vi "strain_test.vi"() -> ()   [LabVIEW 2014]
uses:
  <vilib>/LabVIEW Targets/FPGA/cRIO/shared/nicrio_ModuleControls/nicrio_cRIO-9237_ExcitationVoltageRing.ctl
  <vilib>/LabVIEW Targets/FPGA/cRIO/shared/nicrio_ModuleControls/nicrio_cRIO-9237_DataRatesRing.ctl
  <vilib>/rvi/Emulation/niFpgaGetClockAttributes.vi
  <vilib>/rvi/Emulation/niFpgaSctlEmulationGetInTimedLoop.vi
  <vilib>/rvi/Emulation/niFpgaEmulationReportErrorSimple.vi
  <vilib>/rvi/eio/common/nirviEmuTemplateMethod_errors.vi
  <vilib>/rvi/eio/common/nirviEmuTemplatePropertySet_errors.vi
  <vilib>/rvi/Emulation/niFpgaCriticalErrorInLSC.vi
  <vilib>/eio/EIONode/EIONode.xnode
  <vilib>/rvi/Analysis/measure/butterworth/XNode/niFpgaButterworthFilter.xnode
  <vilib>/eio/EIOPropertyNode/EIOPropertyNode.xnode
  <vilib>/rvi/eio/common/nirviEmuTemplatePropertyGet_errors.vi
  <vilib>/rvi/eio/common/nirviEmuTemplatePropertyGet_noerrors.vi
  <vilib>/rvi/eio/common/nirviEmuTemplatePropertySet_noerrors.vi
panel:
  in  "Offset Cal Enable":bool
  in  "Mod6/Start":bool
  out "Mod1*GF":fxp<+/-,40,9>
  out "Mod1/AI0":fxp<+/-,20,5>
  in  "Data Rate":T1=1 items=["50.000 kS/s (NI 9237)"=1, "25.000 kS/s (NI 9237)"=2, "16.667 kS/s (NI 9237)"=3, "12.500 kS/s (NI 9237)"=4, "10.000 kS/s (NI 9237)"=5, "8.333 kS/s (NI 9237)"=6, "7.143 kS/s (NI 9237)"=7, "6.250 kS/s (NI 9237)"=8, "5.556 kS/s (NI 9237)"=9, "5.000 kS/s (NI 9237)"=10, "4.545 kS/s (NI 9237)"=11, "4.167 kS/s (NI 9237)"=12, "3.846 kS/s (NI 9237)"=13, "3.571 kS/s (NI 9237)"=14, "3.333 kS/s (NI 9237)"=15, "3.125 kS/s (NI 9237)"=16, "2.941 kS/s (NI 9237)"=17, "2.778 kS/s (NI 9237)"=18, "2.632 kS/s (NI 9237)"=19, "2.500 kS/s (NI 9237)"=20, "2.381 kS/s (NI 9237)"=21, "2.273 kS/s (NI 9237)"=22, "2.174 kS/s (NI 9237)"=23, "2.083 kS/s (NI 9237)"=24, "2.000 kS/s (NI 9237)"=25, "1.923 kS/s (NI 9237)"=26, "1.852 kS/s (NI 9237)"=27, "1.786 kS/s (NI 9237)"=28, "1.724 kS/s (NI 9237)"=29, "1.667 kS/s (NI 9237)"=30, "1.613 kS/s (NI 9237)"=31]
  in  "Excitation Voltage":T2=3 items=["2.5 Volts", "3.3 Volts", "5.0 Volts", "10.0 Volts", "External Excitation"]
  in  "Filter switch":bool
  out "Force_s":fxp<+/-,34,15>
  in  "F/S coeff":fxp<+/-,48,15>
  out "Strain":fxp<+/-,36,4>
  in  "Gauge Factor":fxp<+/-,20,4>
  out "Read Data":fxp<+/-,36,4>
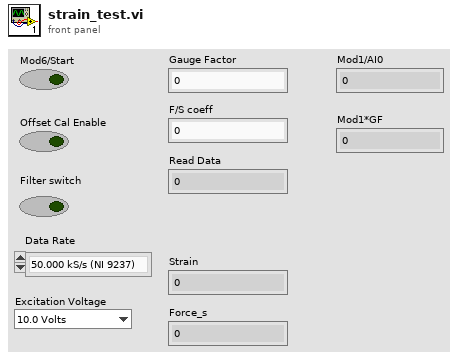
[diagram p1: front panel]
types:
  T1 = typedef "nicrio_cRIO-9237_DataRatesRing.ctl" = u8
  T2 = typedef "nicrio_cRIO-9237_ExcitationVoltageRing.ctl" = u8
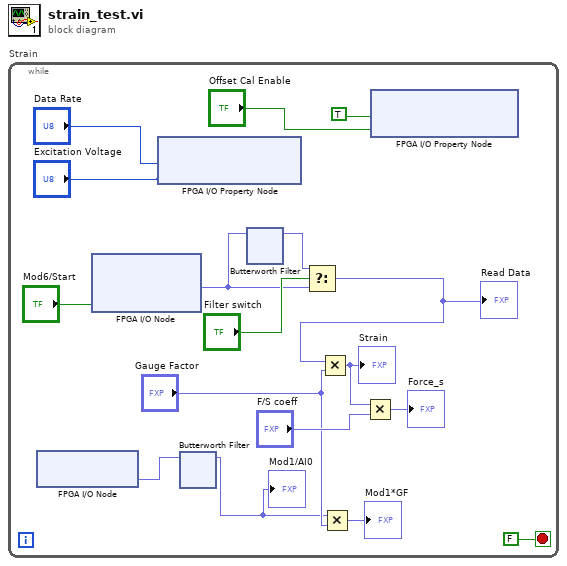
[diagram p0: block diagram]
diagram:
  n1 = while "Strain" {
    stop <- FALSE stop-if-true
    n2 = xnode "FPGA I/O Node"() -> ("Mod1/AI0"=w8:fxp<+/-,20,5>)  [unwired: 1 in, 1 out]
    n3 = xnode "FPGA I/O Node"("Mod6/Start"="Mod6/Start") -> ("Mod6/AI2"=w13:fxp<+/-,24,-4>)  [unwired: 3 in, 3 out]
    n4 = xnode "FPGA I/O Property Node"("Data Rate"="Data Rate", "Excitation Voltage"="Excitation Voltage") -> ()  [unwired: 2 in, 2 out]
    n5 = xnode "Butterworth Filter"("input data"=w8) -> ("output data"=w7:fxp<+/-,24,9>)  [unwired: 2 in]
    "Mod1/AI0" <- w7
    n6 = xnode "Butterworth Filter"("input data"=w13) -> ("output data"=w12:fxp<+/-,28,0>)  [unwired: 2 in]
    n7 = Select(t=w12, s="Filter switch", f=w13) -> (s? t:f=w6:fxp<+/-,28,0>)
    "Read Data" <- w6
    n8 = Multiply(x=w6, y="Gauge Factor") -> (x*y=w17:fxp<+/-,48,4>)
    "Strain" <- w17
    n9 = Multiply(x=w7, y="Gauge Factor") -> (x*y=→"Mod1*GF":fxp<+/-,44,13>)
    n10 = Multiply(x=w17, y="F/S coeff") -> (x*y=→"Force_s":fxp<+/-,64,17>)
    n11 = xnode "FPGA I/O Property Node"("Half-Bridge Enable"=TRUE, "Offset Cal Enable"="Offset Cal Enable") -> ()  [unwired: 2 in, 2 out]
  }
